vi "LRA Test Stand Main.vi"() -> ()   [LabVIEW 2015]
uses:
  Telemetry Packet Type.ctl
  Thermocouple Data.ctl
  Valve Name Enum.ctl
  LaunchPad Communication/Control Packet - Basic.ctl
  Sensors/Sensor Enum.ctl
  Sensors/Transducer Calibration Display.ctl
  Sensors/Transducer Calibration Control.ctl
  Sequence Execution/Sequence State Enum.ctl
  <vilib>/Utility/miscctls.llb/LVRowAndColumnTypeDef.ctl
  System State.ctl
  System State Global Action.ctl
  Valve Button Mapping Global Action.ctl
  Sequence Execution/Test Control Command.ctl
  Valve Port Mapping Action.ctl
  Sensors/Sensor Port Mapping Global Action.ctl
  Sensors/Transducer Calibration Global Action.ctl
  Sequence Execution/Clock Control Enum.ctl
panel:
  out "Sensor Enum":T1
  out "Valve Enum":T2=enum."FV-3"
  in  "Tab Control":T3(tab)
  in  "Abort Test":bool
  in  "Run Test":bool
  in  "NV-2":bool
  in  "OV-4":bool
  in  "OV-3":bool
  in  "OV-2":bool
  in  "FV-4":bool
  in  "FV-3":bool
  in  "FV-2":bool
  in  "Active":bool
  in  "Standby":bool
  in  "Disable":bool
  out "Sequence File":path
  in  "Load Sequence":bool
  out "Log File":path
  out "Mo Pressures":cluster{dbl, dbl, dbl, dbl, dbl}(graph)
  out "Pressures":cluster{dbl, dbl, dbl, dbl, dbl}(graph)
  out "Logging Status":bool
  in  "Stop Recording":bool
  in  "Record":bool
  out "Connection Status":bool
  out "State":bool
  out "Time Display":string
  out "Test Sequence":i32(listbox)
  out "Thermocouple":cluster{dbl, dbl, dbl, dbl, dbl}(graph)
  out "Test State":T4
  out "Array":i32[](array[listbox])
  in  "TD Calibration Control":T5[](array[typedef])
  out "TD Data":T6[](array[typedef]) {"Value" scale=0.0..10.0}
  in  "Sensor Port":u8[](array[numeric])=[0, 1, 2, 3, 4, 5, 6, 7, 8, 9]
  in  "Thermocouple?":bool[](array[boolean])=[TRUE, FALSE, FALSE, TRUE, FALSE, FALSE, FALSE, FALSE, FALSE, FALSE]
  out "Sensor Name":T1[](array[typedef])
  out "Solenoid Commands":bool[](array[boolean])
  in  "Use in Standby":bool[](array[boolean])=[TRUE, FALSE, FALSE, TRUE, FALSE, FALSE, FALSE, FALSE, FALSE, FALSE]
  in  "Solenoid Port":u8[](array[numeric])=[0, 1, 2, 3, 4, 5, 6, 7, 8, 9]
  out "Valve Name":T2[](array[typedef])
  out "TC 4":T7
  out "TC 3":T7
  out "TC 2":T7
  out "TC 1":T7
  out "TC 0":T7
  in  "TD Reference Voltage \n(5V Nominal)":dbl format="%.3g"
  out "Telemetry Packet":T8
  out "Command Packet":T9
  in  "Man Sol 7":bool
  in  "Man Sol 6":bool
  in  "Man Sol 5":bool
  in  "Man Sol 4":bool
  in  "Man Sol 3":bool
  in  "Man Sol 2":bool
  in  "Man Sol 1":bool
  in  "Man Sol 0":bool
  # "look a  diagram with a bunch of status things goes here"
  # "State Control"
  # "Sensor Calibration"
  # "Thermocouple Data"
  # "Valve Configuration"
  # "Sensor Configuration"
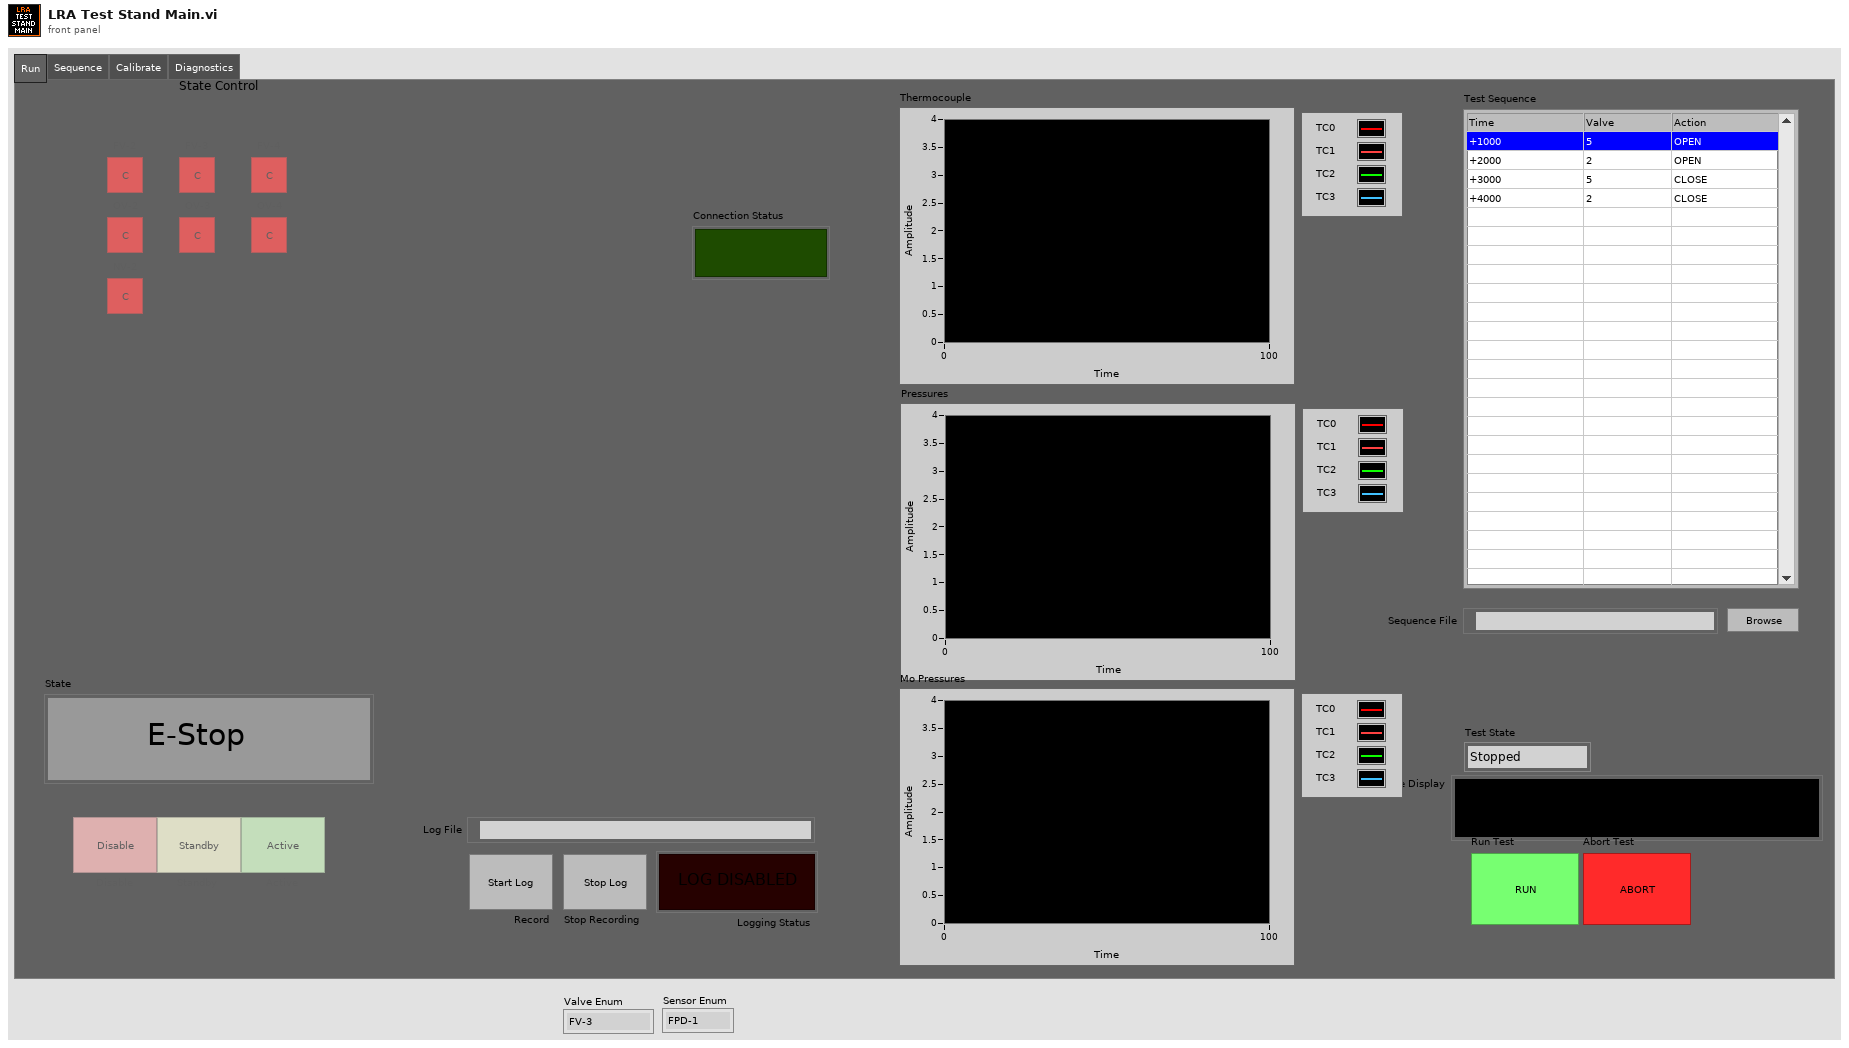
[diagram p1: front panel]
types:
  T1 = typedef "Sensor Enum.ctl" = enum16{"FPD-1", "OPD-1", "FPD-2", "OPD-2"}
  T2 = typedef "Valve Name Enum.ctl" = enum16{"FV-4", "FV-3", "FV-2", "OV-4", "OV-3", "OV-2", "NV-2"}
  T3 = enum32{"Run", "Sequence", "Calibrate", "Diagnostics"}
  T4 = typedef "Sequence State Enum.ctl" = enum16{"Stopped", "Start", "Running", "Abort", "End"}
  T5 = typedef "Transducer Calibration Control.ctl" = cluster{"Scale":dbl, "Offset":dbl}
  T6 = typedef "Transducer Calibration Display.ctl" = cluster{"Value":dbl, "Raw":dbl, "Scaled":dbl, "Sensor Name":T1, "Port":u32}
  T7 = typedef "Thermocouple Data.ctl" = cluster{"TC Temp":dbl, "Internal Temp":dbl, "Fault":bool, "Short to VCC":bool, "Short to GND":bool, "Open Circuit":bool}
  T8 = typedef "Telemetry Packet Type.ctl" = cluster{"Timestamp\n":u32, "Transducer Value":u16[], "Main Loop Rate":u32, "Solenoid State":bool[], "Output Enabled":bool, "Solenoids Powered":bool, "TC Data":T7[], "TD Rate":u32, "TD Execution Time":u32, "TC Rate":u32, "TC Execution Time":u32}
  T9 = typedef "Control Packet - Basic.ctl" = cluster{"Solenoid Commands":bool[], "Output Enable":bool, "Timestamp":u32}
  T10 = typedef "Test Control Command.ctl" = enum16{"Get Notifier", "Init", "Start", "Stop"}
  T11 = typedef "Valve Button Mapping Global Action.ctl" = enum16{"Get", "Set"}
  T12 = typedef "System State Global Action.ctl" = enum16{"Get", "Set", "Initialize"}
  T13 = typedef "System State.ctl" = enum16{"Disabled", "E-Stop", "Standby", "Active"}
  T14 = typedef "LVRowAndColumnTypeDef.ctl" = cluster{"Row":i32, "Column":i32}
  T15 = typedef "Clock Control Enum.ctl" = enum16{"Set", "Get", "Start", "Stop"}
  T16 = typedef "Transducer Calibration Global Action.ctl" = enum16{"Get", "Set"}
  T17 = typedef "Sensor Port Mapping Global Action.ctl" = enum16{"Get", "Set"}
  T18 = typedef "Valve Port Mapping Action.ctl" = enum16{"Get", "Set"}
  T19 = typedef "Single Test Sequence.ctl" = cluster{"Actions":T20[], "Triggers":T22[], "Name":string}
  T20 = typedef "Test Sequence Action.ctl" = cluster{"Time":i32, "Action":T21, "Valve":T2}
  T21 = typedef "Valve Action Enum.ctl" = enum16{"Open", "Close"}
  T22 = typedef "Test Sequence Trigger.ctl" = cluster{"Sensor":T1, "Begin Time (ms)":dbl, "End Time(ms)":dbl, "Min Value":dbl, "Max Value":dbl}
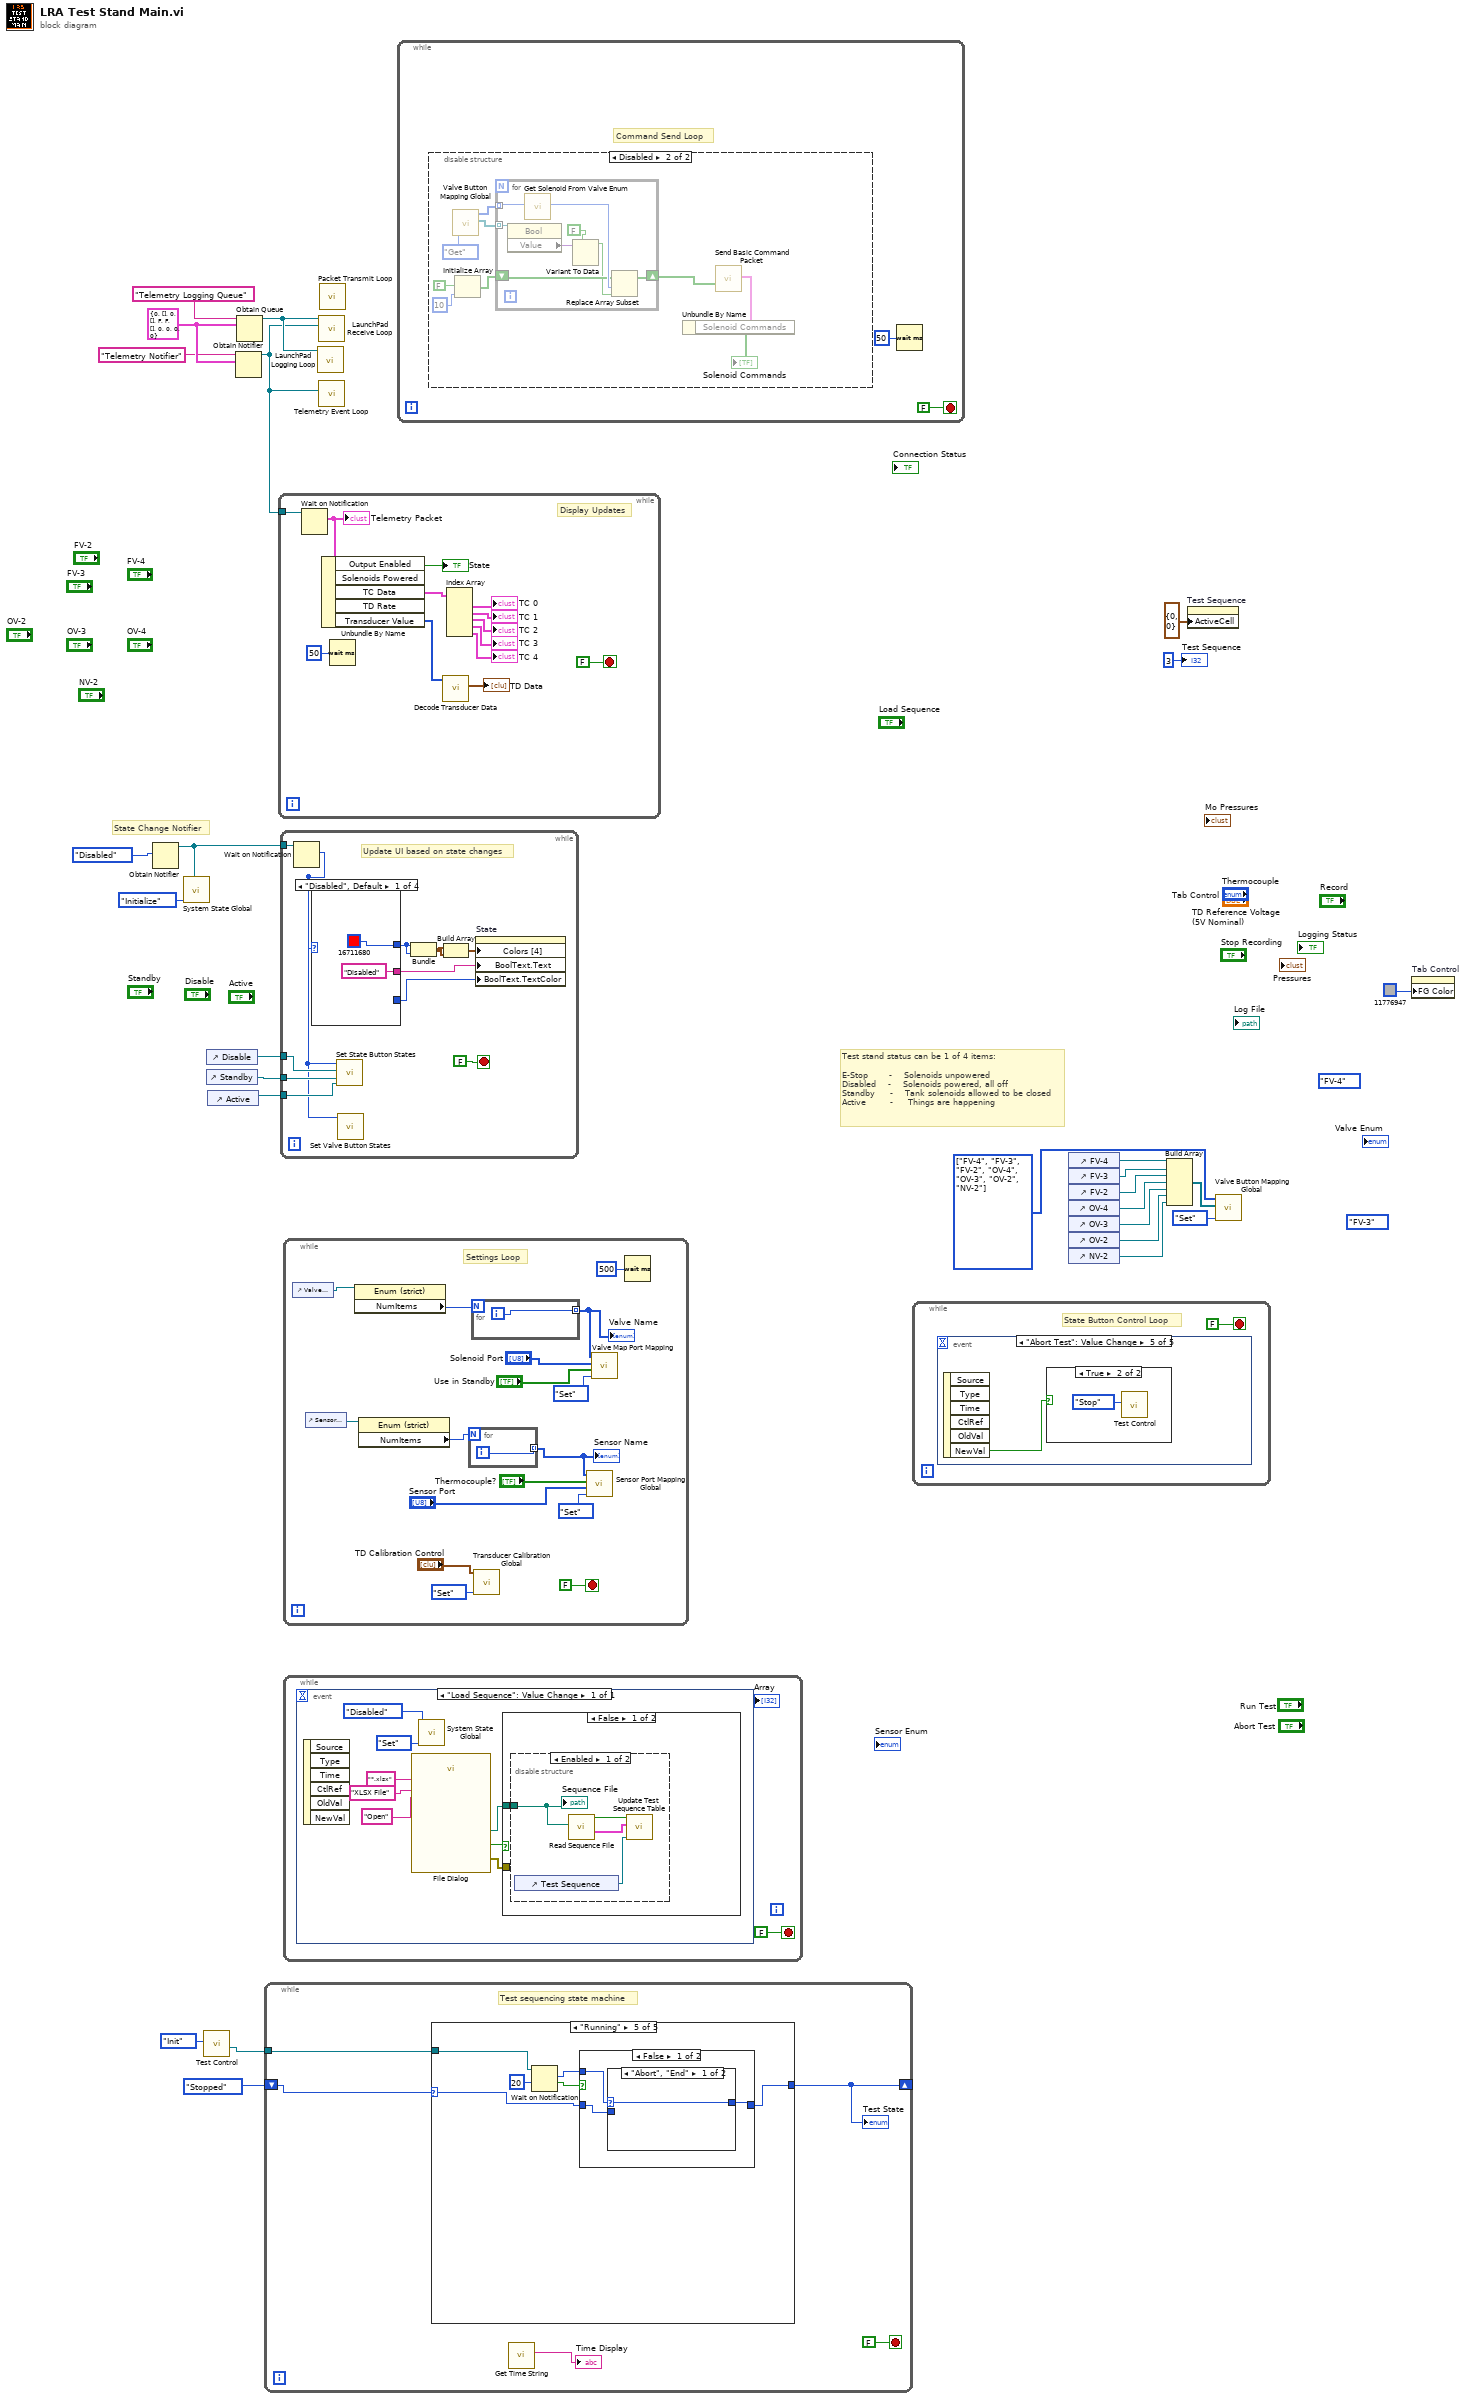
[diagram p0: block diagram]
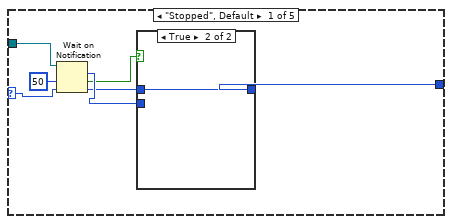
[diagram p2: hidden frame]
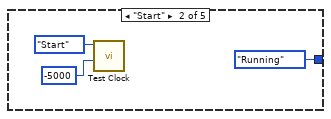
[diagram p5: hidden frame]
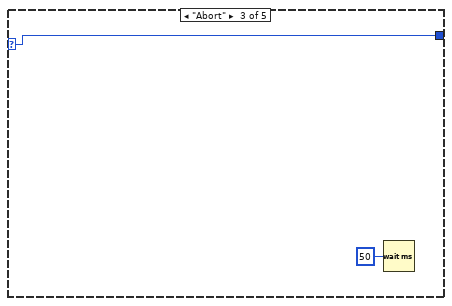
[diagram p6: hidden frame]
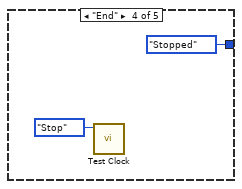
[diagram p7: hidden frame]
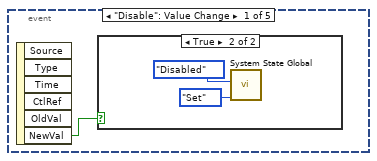
[diagram p10: hidden frame]
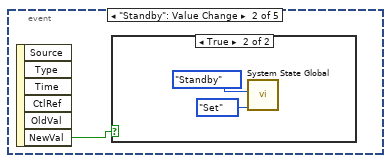
[diagram p12: hidden frame]
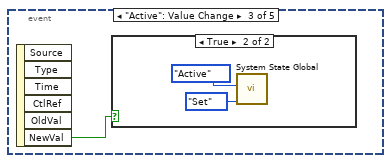
[diagram p14: hidden frame]
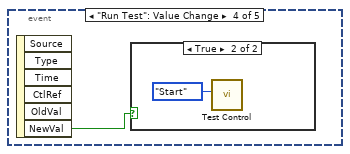
[diagram p16: hidden frame]
diagram:
  w5 = T2[] [enum."FV-4", enum."FV-3", enum."FV-2", enum."OV-4", enum."OV-3", enum."OV-2", enum."NV-2"] items=["FV-4", "FV-3", "FV-2", "OV-4", "OV-3", "OV-2", "NV-2"] ("Valve Name")
  (unwired) Valve_Name_Enum."FV-4" ("Enum")
  (unwired) Valve_Name_Enum."FV-3" ("Enum")
  w25 = T8 {"Timestamp\n"=0, "Transducer Value"=[], "Main Loop Rate"=0, "Solenoid State"=[], "Output Enabled"=FALSE, "Solenoids Powered"=FALSE, "TC Data"=[], "TD Rate"=0, "TD Execution Time"=0, "TC Rate"=0, "TC Execution Time"=0} ("Cluster")
  # "State Change Notifier"
  # "Test stand status can be 1 of 4 items:\n\nE-Stop       -    Solenoids unpowered\nDisabled    -    Solenoids powered, all off\nStandby     -    Tank solenoids allowed to be closed\nActive        -     Things are happening"
  n1 = Obtain Notifier(notification data type=System_State."Disabled" ("State")) -> (notifier out=w20:refnum<notifier>)  [unwired: 3 in, 2 out]
  n2 = call "System State Global.vi"("Notifier In"=w20, "Action"=System_State_Global_Action."Initialize") -> ()  [unwired: 8 in, 2 out]
  n3 = call "Test Control.vi"("Command"=Test_Control_Command."Init") -> ("notifier out"=w1:refnum<notifier>)  [unwired: 10 in]
  n4 = control-ref of="Disable"() -> (w17:refnum<vi>)
  n5 = control-ref of="Standby"() -> (w16:refnum<vi>)
  n6 = control-ref of="Active"() -> (w15:refnum<vi>)
  n7 = Obtain Notifier(name (unnamed)="Telemetry Notifier", notification data type=w25) -> (notifier out=w18:refnum<notifier>)  [unwired: 2 in, 2 out]
  n8 = Obtain Queue(name (unnamed)="Telemetry Logging Queue", element data type=w25) -> (queue out=w26:refnum<queue>)  [unwired: 3 in, 2 out]
  n9 = while {
    shift-right: [w31] -> _
    shift-left: Sequence_State_Enum."Stopped" -> [w30]
    tunnel: w1 -> [w28]
    stop <- FALSE stop-if-true
    # "Test sequencing state machine"
    n10 = case shown="\"Running\"" w30 {
      selector: w30 -> [w36 _ w49 _ w55]
      tunnel: [w37 Sequence_State_Enum."Running" w49 Sequence_State_Enum."Stopped" w54] -> w31
      tunnel: w28 -> [w33 _ _ _ w52]
      frame "Stopped", Default {
        n11 = Wait on Notification(notifier=w33, timeout in ms (-1)=50) -> (notification=w38:T4, timed out?=w34:bool)  [unwired: 2 in, 2 out]
        n12 = case shown="True" w34 {
          tunnel: w38 -> [w41 _]
          tunnel: [w40 w44] -> w37
          tunnel: w36 -> [w39 w44]
          frame False {
            n13 = case shown="\"Stopped\", Default" w41 {
              selector: w41 -> [_ w43]
              tunnel: [w42 w43] -> w40
              tunnel: w39 -> [w42 _]
              frame "Stopped", Default {
              }
              frame "Start" {
              }
            }
          }
          frame True {
          }
        }
      }
      frame "Start" {
        n14 = call "Test Clock.vi"("Set Time"=-5000, "Command"=Clock_Control_Enum."Start") -> ()  [unwired: 8 in, 2 out]
      }
      frame "Abort" {
        n15 = Wait (ms)(milliseconds to wait=u32 50) -> ()  [unwired: 1 out]
      }
      frame "End" {
        n16 = call "Test Clock.vi"("Command"=Clock_Control_Enum."Stop") -> ()  [unwired: 9 in, 2 out]
      }
      frame "Running" {
        n17 = Wait on Notification(notifier=w52, timeout in ms (-1)=20) -> (notification=w53:T4, timed out?=w56:bool)  [unwired: 2 in, 2 out]
        n18 = case shown="False" w56 {
          tunnel: w55 -> [w58 w63]
          tunnel: [w59 w63] -> w54
          tunnel: w53 -> [w60 _]
          frame False {
            n19 = case shown="\"Abort\", \"End\"" w60 {
              selector: w60 -> [w61 _]
              tunnel: [w61 w62] -> w59
              tunnel: w58 -> [_ w62]
              frame "Abort", "End" {
              }
              frame Default {
              }
            }
          }
          frame True {
          }
        }
      }
    }
    "Test State" <- w31
    n20 = call "Get Time String.vi"() -> ("Time String"=→"Time Display":string)  [unwired: 11 in]
  }
  n21 = while {
    tunnel: w18 -> [w76]
    stop <- FALSE stop-if-true
    # "Display Updates"
    n22 = Wait on Notification(notifier=w76) -> (notification=w73:T8)  [unwired: 3 in, 3 out]
    "Telemetry Packet" <- w73
    n23 = Unbundle By Name(w73) -> ("Output Enabled"=→"State":bool, "TC Data"=w71:T7[], "Transducer Value"=w65:u16[])  [unwired: 2 out]
    n24 = Wait (ms)(milliseconds to wait=u32 50) -> ()  [unwired: 1 out]
    n25 = call "Decode Transducer Data.vi"("Transducer Value"=w65) -> ("TD Data"=→"TD Data":T6[])  [unwired: 10 in]
    n26 = Index Array(array=w71) -> (element #1=→"TC 0":T7, element #2=→"TC 1":T7, element #3=→"TC 2":T7, element #4=→"TC 3":T7, element #5=→"TC 4":T7)  [unwired: 5 in]
  }
  n27 = while {
    tunnel: w20 -> [w87]
    tunnel: w17 -> [w81]
    tunnel: w16 -> [w80]
    tunnel: w15 -> [w79]
    stop <- FALSE stop-if-true
    # "Update UI based on state changes"
    n28 = Wait on Notification(notifier=w87) -> (notification=w78:T13)  [unwired: 3 in, 3 out]
    n29 = case shown="\"Disabled\", Default" w78 {
      tunnel: ["Disabled" ("Boolean Text.Text") "E-Stop" ("Boolean Text.Text") "Standby" ("Boolean Text.Text") "Active" ("Boolean Text.Text")] -> w85
      tunnel: [u32 16711680 u32 10066329 u32 16773906 u32 6618880] -> w82
      tunnel: [_ u32 0 _ _] -> w77
      frame "Disabled", Default {
      }
      frame "E-Stop" {
      }
      frame "Standby" {
      }
      frame "Active" {
      }
    }
    n30 = call "Set State Button States.vi"("Active"=w79, "Standby"=w80, "Disable"=w81, "State"=w78) -> ()  [unwired: 8 in]
    n31 = call "Set Valve Button States.vi"("State"=w78) -> ()  [unwired: 11 in]
    n32 = Bundle(w82, w82) -> (w84:cluster{u32, u32})  [unwired: 1 in]
    n33 = Build Array(w84, w84) -> (w83:cluster{u32, u32}[])
    n34 = property on="State" class="Bool (strict)"("Colors [4]"=w83, "BoolText.Text"=w85, "BoolText.TextColor"=w77) -> ()  [unwired: 2 in, 2 out]
  }
  n35 = while {
    stop <- FALSE stop-if-true
    # "Settings Loop"
    n36 = control-ref of="Valve Enum"() -> (w112:refnum<vi>)
    n37 = control-ref of="Sensor Enum"() -> (w104:refnum<vi>)
    n38 = property class="Enum (strict)"(reference=w112) -> ("NumItems"=w111:u32)  [unwired: 1 in, 2 out]
    n39 = property class="Enum (strict)"(reference=w104) -> ("NumItems"=w103:u32)  [unwired: 1 in, 2 out]
    n40 = for {
      N: w103 -> [_]
      tunnel: [w113] -> w99 mode=indexing
      i -> [w113]
    }
    "Sensor Name" <- w99
    n41 = for {
      N: w111 -> [_]
      tunnel: [w114] -> w110 mode=indexing
      i -> [w114]
    }
    "Valve Name" <- w110
    n42 = call "Transducer Calibration Global.vi"("Action"=Transducer_Calibration_Global_Action."Set", "Data In"="TD Calibration Control") -> ()  [unwired: 9 in, 1 out]
    n43 = call "Sensor Port Mapping Global.vi"("Action"=Sensor_Port_Mapping_Global_Action."Set", "Ports"="Sensor Port", "Thermocouple?"="Thermocouple?", "Sensors"=w99) -> ()  [unwired: 7 in, 1 out]
    n44 = call "Valve Map Port Mapping.vi"("Action"=Valve_Port_Mapping_Action."Set", "Allowed In Standby?"="Use in Standby", "Solenoid Port List"="Solenoid Port", "Valve List"=w110) -> ()  [unwired: 7 in, 1 out]
    n45 = Wait (ms)(milliseconds to wait=u32 500) -> ()  [unwired: 1 out]
  }
  n46 = while {
    stop <- FALSE stop-if-true
    n47 = event shown="[0] \"Load Sequence\": Value Change" {
      selector: _ -> [_]
      dyn-events: _ -> [_]
      timeout: _ -> [_]
      event "Load Sequence": Value Change {
        n48 = event-data() -> ()  [unwired: 1 in, 6 out]
        n49 = call "File Dialog"("button label"="Open", "pattern (all files)"="*.xlsx", "pattern label"="XLSX File") -> ("selected path"=w119:path, "cancelled"=w120:bool, "error out"=w118:errorcluster)  [unwired: 9 in, 1 out]
        n50 = call "System State Global.vi"("Action"=System_State_Global_Action."Set", "State In"=System_State."Disabled") -> ()  [unwired: 8 in, 2 out]
        n51 = case shown="False" w120 {
          tunnel: w119 -> [w124 _]
          tunnel: w118 -> [_ _]
          frame False {
            n52 = disable-structure shown="Enabled" {
              disable-tunnel: w124 -> [w128 _]
              frame Enabled {
                n53 = control-ref of="Test Sequence"() -> (w126:refnum<vi>)
                n54 = call "Read Sequence File.vi"("Path"=w128) -> ("Test Sequence"=w125:T19[], "Valid?"=w127:bool)  [unwired: 9 in]
                n55 = call "Update Test Sequence Table.vi"("Listbox Reference"=w126, "Test Sequence"=w125, "Valid?"=w127) -> ()  [unwired: 9 in]
                "Sequence File" <- w128
              }
              frame Disabled {
              }
            }
          }
          frame True {
          }
        }
      }
    }
  }
  n56 = call "LaunchPad Logging Loop.vi"("Queue in"=w26) -> ()  [unwired: 11 in]
  n57 = call "LaunchPad Receive Loop.vi"("Telemetry Notifier Ref"=w18, "Telemetry Queue Ref"=w26) -> ()  [unwired: 10 in]
  n58 = call "Telemetry Event Loop.vi"("Telemetry Notifier"=w18) -> ()  [unwired: 11 in]
  n59 = call "Packet Transmit Loop.vi"() -> ()  [unwired: 12 in]
  n60 = while {
    stop <- FALSE stop-if-true
    # "Command Send Loop"
    n61 = disable-structure shown="Disabled" {
      frame Enabled {
        n62 = call "System State Global.vi"("Action"=System_State_Global_Action."Get") -> ("State Out"=w137:T13)  [unwired: 9 in, 1 out]
        n63 = Build Array("Man Sol 0", "Man Sol 1", "Man Sol 2", "Man Sol 3", "Man Sol 4", "Man Sol 5", "Man Sol 6", "Man Sol 7") -> (w139:bool[])
        n64 = Equal?(x=System_State."Active" ("y"), y=w137) -> (x = y?=w134:bool)
        n65 = Equal?(x=System_State."Standby" ("y"), y=w137) -> (x = y?=w133:bool)
        n66 = Or(x=w134, y=w133) -> ()  [unwired: 1 out]
        n67 = call "Send Basic Command Packet.vi"("Solenoid States"=w139, "Output Enable"=TRUE) -> ("Built Packet"=→"Command Packet":T9)  [unwired: 9 in]
      }
      frame Disabled {
        n68 = call "Valve Button Mapping Global.vi"("Action"=Valve_Button_Mapping_Global_Action."Get") -> ("Buttons"=w155:refnum<vi>[], "Valves"=w156:T2[])  [unwired: 9 in]
        n69 = Initialize Array(FALSE, 10 ("dimension size")) -> (w150:bool[])
        n70 = for {
          tunnel: w156 -> [w161] mode=indexing
          tunnel: w155 -> [w164] mode=indexing
          shift-right: [w158] -> w154
          shift-left: w150 -> [w159]
          n71 = property class="Bool"(reference=w164) -> ("Value"=w163:variant)  [unwired: 1 in, 2 out]
          n72 = call "Get Solenoid From Valve Enum.vi"("Valve"=w161) -> ("Port"=w160:u8)  [unwired: 9 in, 1 out]
          n73 = Variant To Data(type=FALSE, Variant=w163) -> (data=w157:bool)  [unwired: 1 in, 1 out]
          n74 = Replace Array Subset(array=w159, new element=w157, index=w160) -> (w158:bool[])
        }
        n75 = call "Send Basic Command Packet.vi"("Solenoid States"=w154) -> ("Built Packet"=w153:T9)  [unwired: 10 in]
        n76 = Unbundle By Name(w153) -> ("Solenoid Commands"=→"Solenoid Commands":bool[])
      }
    }
    n77 = Wait (ms)(milliseconds to wait=u32 50) -> ()  [unwired: 1 out]
  }
  n78 = while {
    stop <- FALSE stop-if-true
    # "State Button Control Loop"
    n79 = event shown="[4] \"Abort Test\": Value Change" {
      selector: _ -> [_ _ _ _ _]
      dyn-events: _ -> [_ _ _ _ _]
      timeout: _ -> [_ _ _ _ _]
      event "Disable": Value Change {
        n80 = event-data() -> ("NewVal"=w166:bool)  [unwired: 1 in, 5 out]
        n81 = case shown="True" w166 {
          frame False {
          }
          frame True {
            n82 = call "System State Global.vi"("Action"=System_State_Global_Action."Set", "State In"=System_State."Disabled") -> ()  [unwired: 8 in, 2 out]
          }
        }
      }
      event "Standby": Value Change {
        n83 = event-data() -> ("NewVal"=w169:bool)  [unwired: 1 in, 5 out]
        n84 = case shown="True" w169 {
          frame False {
          }
          frame True {
            n85 = call "System State Global.vi"("Action"=System_State_Global_Action."Set", "State In"=System_State."Standby") -> ()  [unwired: 8 in, 2 out]
          }
        }
      }
      event "Active": Value Change {
        n86 = event-data() -> ("NewVal"=w172:bool)  [unwired: 1 in, 5 out]
        n87 = case shown="True" w172 {
          frame False {
          }
          frame True {
            n88 = call "System State Global.vi"("Action"=System_State_Global_Action."Set", "State In"=System_State."Active") -> ()  [unwired: 8 in, 2 out]
          }
        }
      }
      event "Run Test": Value Change {
        n89 = event-data() -> ("NewVal"=w175:bool)  [unwired: 1 in, 5 out]
        n90 = case shown="True" w175 {
          frame False {
          }
          frame True {
            n91 = call "Test Control.vi"("Command"=Test_Control_Command."Start") -> ()  [unwired: 10 in, 1 out]
          }
        }
      }
      event "Abort Test": Value Change {
        n92 = event-data() -> ("NewVal"=w177:bool)  [unwired: 1 in, 5 out]
        n93 = case shown="True" w177 {
          frame False {
          }
          frame True {
            n94 = call "Test Control.vi"("Command"=Test_Control_Command."Stop") -> ()  [unwired: 10 in, 1 out]
          }
        }
      }
    }
  }
  n95 = control-ref of="FV-4"() -> (w14:refnum<vi>)
  n96 = control-ref of="FV-3"() -> (w13:refnum<vi>)
  n97 = control-ref of="FV-2"() -> (w12:refnum<vi>)
  n98 = control-ref of="OV-4"() -> (w11:refnum<vi>)
  n99 = control-ref of="OV-3"() -> (w10:refnum<vi>)
  n100 = control-ref of="OV-2"() -> (w9:refnum<vi>)
  n101 = control-ref of="NV-2"() -> (w8:refnum<vi>)
  n102 = Build Array(w14, w13, w12, w11, w10, w9, w8) -> (w6:refnum<vi>[])
  n103 = property on="Test Sequence" class="MCListbox (strict)"("ActiveCell"=T14 {"Row"=0, "Column"=0} ("Active Cell:Active Cell")) -> ()  [unwired: 2 in, 2 out]
  n104 = call "Valve Button Mapping Global.vi"("Action"=Valve_Button_Mapping_Global_Action."Set", "Valve Buttons"=w6, "Valves"=w5) -> ()  [unwired: 7 in, 2 out]
  n105 = property on="Tab Control" class="TabCtl (strict)"("FG Color"=u32 11776947) -> ()  [unwired: 2 in, 2 out]
  "Test Sequence" <- 3 ("Test Sequence")
